vi "Draw_Segment_at_Coords.vi"(8 "error in (no error)":errorcluster, 9 "Cage type":T1 items=["Round", "Square", "Donut-maze", "T-maze", "Sociability maze", ""], 10 "Image Drawing Parameters":T6, 11 "Refnum in":T7) -> (0 "error out":errorcluster, 3 "Refnum out":T7)   [LabVIEW 2018, in "Cage Diagram.lvlib"]
uses:
  Cage Diagram.lvlib
  <vilib>/vision/Image Controls.llb/IMAQ Image.ctl
  SubVi's/Controls/CTL_Segments_Colors_(pie).ctl
  Common_Resources.lvlib
  Typedefs/CTL_Image_Scaling_info.ctl
  Typedefs/CTL_Cage_dimensions.ctl
  SubVi's/Controls/CTL_Draw_Area_Size.ctl
  Typedefs/CTL_Cage_type.ctl
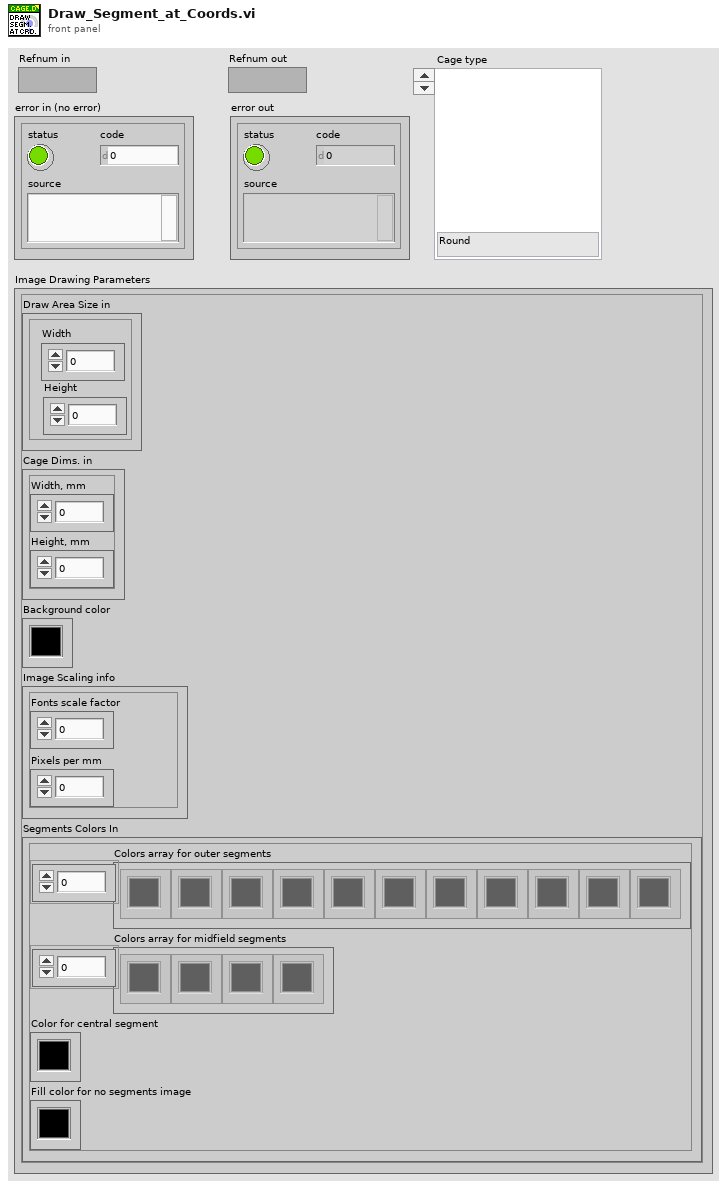
[diagram p1: front panel]
types:
  T1 = typedef "Cage Diagram.lvlib/CTL_Cage_type.ctl" = u16
  T2 = typedef "Common_Resources.lvlib/CTL_Draw_Area_Size.ctl" = cluster{"Width":i32, "Height":i32}
  T3 = typedef "Cage Diagram.lvlib/CTL_Cage_dimensions.ctl" = cluster{"Width, mm":dbl, "Height, mm":dbl}
  T4 = typedef "Cage Diagram.lvlib/CTL_Image_Scaling_info.ctl" = cluster{"Fonts scale factor":dbl, "Pixels per mm":dbl}
  T5 = typedef "Common_Resources.lvlib/CTL_Segments_Colors_(pie).ctl" = cluster{"Colors array for outer segments":u32[], "Colors array for midfield segments":u32[], "Color for central segment":u32, "Fill color for no segments image":u32}
  T6 = cluster{"Draw Area Size in":T2, "Cage Dims. in":T3, "Background color":u32, "Image Scaling info":T4, "Segments Colors In":T5}
  T7 = typedef "IMAQ Image.ctl" = refnum<image>
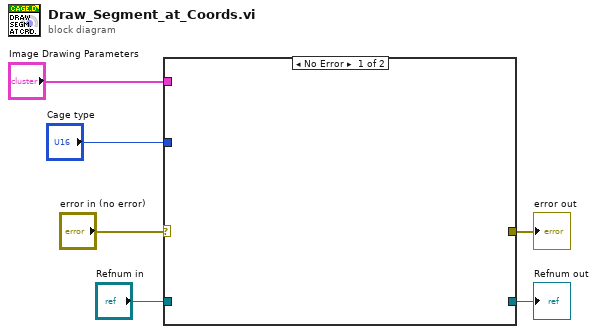
[diagram p0: block diagram]
diagram:
  n1 = case shown="No Error" "error in (no error)" {
    selector: "error in (no error)" -> [_ w8]
    tunnel: [_ w8] -> w5
    tunnel: "Refnum in" -> [_ w7]
    tunnel: "Image Drawing Parameters" -> [_ _]
    tunnel: [_ w7] -> w2
    tunnel: "Cage type" -> [_ _]
    frame No Error {
    }
    frame Error {
    }
  }
  "Refnum out" <- w2
  "error out" <- w5
